vi "Default Instrument Setup.vi"(8 "error in (no error)":errorcluster, 11 "VISA resource name":refnum<visa-resource-name>) -> (0 "error out":errorcluster, 3 "VISA resource name out":refnum<visa-resource-name>)   [LabVIEW 2020, in "QuPMXdriver.lvlib"]
doc: "Sends a default command string to the instrument whenever a new VISA session is opened, or the instrument is reset. Use this VI as a subVI for the <b>Initialize</b> and <b>Reset</b> VIs. Altering this VI could cause these two VIs to operate incorrectly."
uses:
  QuPMXdriver.lvlib
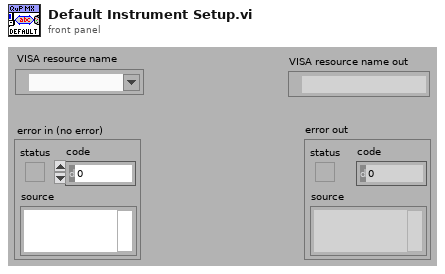
[diagram p1: front panel]
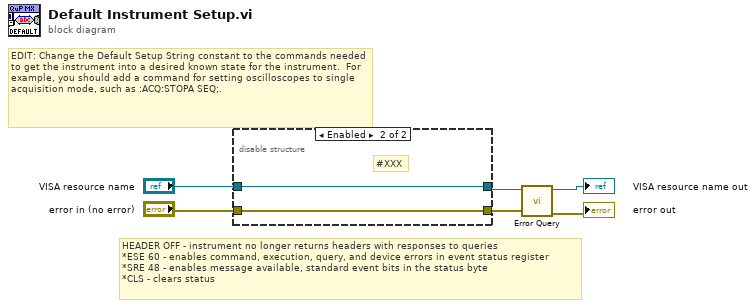
[diagram p0: block diagram]
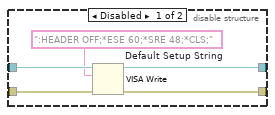
[diagram p2: hidden frame]
diagram:
  # "HEADER OFF - instrument no longer returns headers with responses to queries\n*ESE 60 - enables command, execution, query, and device errors in event status register\n*SRE 48 - enables message available, standard event bits in the status byte\n*CLS - clears status"
  # "EDIT: Change the Default Setup String constant to the commands needed to get the instrument into a desired known state for the instrument.  For example, you should add a command for setting oscilloscopes to single acquisition mode, such as :ACQ:STOPA SEQ;."
  n1 = disable-structure shown="Enabled" {
    disable-tunnel: "VISA resource name" -> [w11 w13]
    disable-tunnel: "error in (no error)" -> [w10 w12]
    disable-tunnel: [w9 w13] -> w1
    disable-tunnel: [w8 w12] -> w4
    frame Disabled {
      w7 = ":HEADER OFF;*ESE 60;*SRE 48;*CLS;"  # Default Setup String
      n2 = VISA Write(VISA resource name=w11, write buffer=w7, error in (no error)=w10) -> (VISA resource name out=w9:refnum<visa-resource-name>, error out=w8:errorcluster)  [unwired: 1 out]
    }
    frame Enabled {
      # "#XXX"
    }
  }
  n3 = call "Error Query.vi"("error in (no error)"=w4, "VISA resource name"=w1) -> ("error out"=→"error out":errorcluster, "VISA resource name out"=→"VISA resource name out":refnum<visa-resource-name>)  [unwired: 8 in]
